vi "Xbox Controller Cluster Output 6740.vi"(11 "Joystick Name":string="Xbox") -> (0 "Buttons":T1, 3 "Axis":T2, 4 "POVs":i16[](array[numeric]))   [LabVIEW 2020]
uses:
  <vilib>/Rock Robotics/WPI/Utilities/WPI_GetSetVariantRefNum.vi
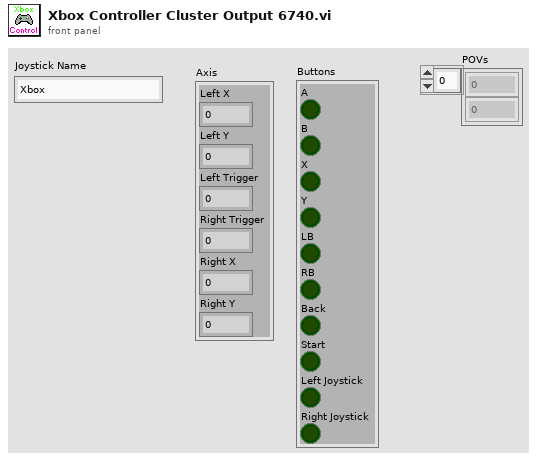
[diagram p1: front panel]
types:
  T1 = cluster{"A":bool, "B":bool, "X":bool, "Y":bool, "LB":bool, "RB":bool, "Back":bool, "Start":bool, "Left Joystick":bool, "Right Joystick":bool}
  T2 = cluster{"Left X":dbl, "Left Y":dbl, "Left Trigger":dbl, "Right Trigger":dbl, "Right X":dbl, "Right Y":dbl}
  T3 = typedef "WPI_JoystickDevRef.ctl" = cluster{"Device":T4}
  T4 = typedef "WPI_JoystickDeviceEnum.ctl" = enum16{"USB 0", "USB 1", "USB 2", "USB 3", "USB 4", "USB 5"}
  T5 = cluster{"Axes[0]":dbl, "Axes[1]":dbl, "Axes[2]":dbl, "Axes[3]":dbl, "Axes[4]":dbl, "Axes[5]":dbl, "Axes[6]":dbl, "Axes[7]":dbl, "Axes[8]":dbl}
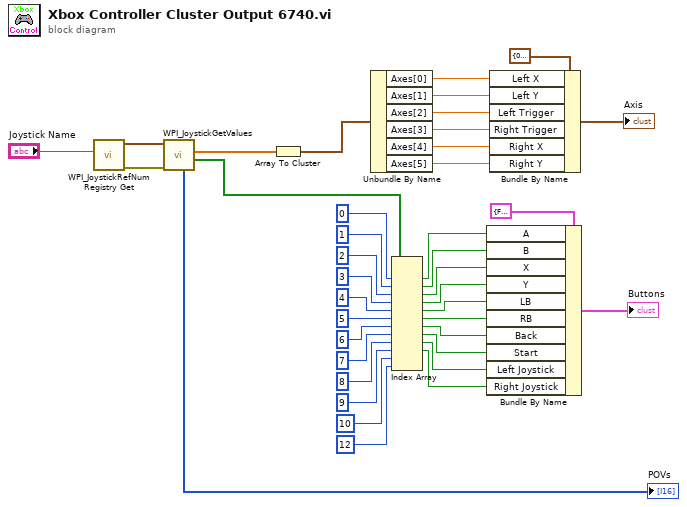
[diagram p0: block diagram]
diagram:
  n1 = call <vilib>:"WPI_JoystickRefNum Registry Get.vi"("refnum name"="Joystick Name") -> ("error out"=w1:errorcluster, "JoystickDevRef"=w30:T3)  [unwired: 9 in]
  n2 = call <vilib>:"WPI_JoystickGetValues.vi"("error in (no error)"=w1, "JoystickDevRef"=w30) -> ("Buttons"=w28:bool[], "Axes"=w4:dbl[], "POVs"=→"POVs":i16[])  [unwired: 5 in, 2 out]
  n3 = Array To Cluster(array=w4) -> (cluster=w3:T5)
  n4 = Unbundle By Name(w3) -> ("Axes[0]"=w38:dbl, "Axes[1]"=w37:dbl, "Axes[2]"=w36:dbl, "Axes[3]"=w35:dbl, "Axes[4]"=w34:dbl, "Axes[5]"=w33:dbl)
  n5 = Index Array(array=w28, index #1=0 ("index"), index #2=1 ("index"), index #3=2 ("index"), index #4=3 ("index"), index #5=4 ("index"), index #6=5 ("index"), index #7=6 ("index"), index #8=7 ("index"), index #9=8 ("index"), index #10=9 ("index"), index #11=10 ("index"), index #12=12 ("index")) -> (element #1=w14:bool, element #2=w13:bool, element #3=w12:bool, element #4=w11:bool, element #5=w10:bool, element #6=w9:bool, element #7=w8:bool, element #8=w7:bool, element #9=w6:bool, element #10=w5:bool)  [unwired: 2 out]
  n6 = Bundle By Name(cluster=T1 {"A"=FALSE, "B"=FALSE, "X"=FALSE, "Y"=FALSE, "LB"=FALSE, "RB"=FALSE, "Back"=FALSE, "Start"=FALSE, "Left Joystick"=FALSE, "Right Joystick"=FALSE} ("input cluster"), "A"=w14, "B"=w13, "X"=w12, "Y"=w11, "LB"=w10, "RB"=w9, "Back"=w8, "Start"=w7, "Left Joystick"=w6, "Right Joystick"=w5) -> (→"Buttons":T1)
  n7 = Bundle By Name(cluster=T2 {"Left X"=0.0, "Left Y"=0.0, "Left Trigger"=0.0, "Right Trigger"=0.0, "Right X"=0.0, "Right Y"=0.0} ("input cluster"), "Left X"=w38, "Left Y"=w37, "Left Trigger"=w36, "Right Trigger"=w35, "Right X"=w34, "Right Y"=w33) -> (→"Axis":T2)
